vi "2DROISpectrum.vi"(4 "Zero Pad?":bool, 6 "convert output to dB?":bool, 7 "FFT size":u16(ring) items=["next 2^n", "8", "16", "32", "64", "128", "256", "512"], 8 "Cal File":dbl[](array[numeric]) format="%.2f", 9 "Array Subset":T1 {"length of y" format="%.2f"; "y start" format="%.2f"; "length of x" format="%.2f"; "x start" format="%.2f"}, 10 "freq (MHz)":dbl format="%.2f", 11 "2-D data array":i16[][](array[numeric])) -> (0 "Length of padded array":i32, 1 "df (MHz)":dbl format="%.2f", 3 "power spectrum in dB":dbl[][](array[numeric]) format="%.2f")   [LabVIEW 2022 SP3]
uses:
  <vilib>/Analysis/4window.llb/Hamming Window (DBL).vi
  <vilib>/Analysis/2dsp.llb/Real FFT.vi
  <vilib>/Analysis/2dsp.llb/Complex FFT.vi
  <vilib>/Analysis/4window.llb/AllCosWindow (DBL).vi
  <vilib>/Analysis/NI_AALPro.lvlib
panel:
  # "Columns represent scan line"
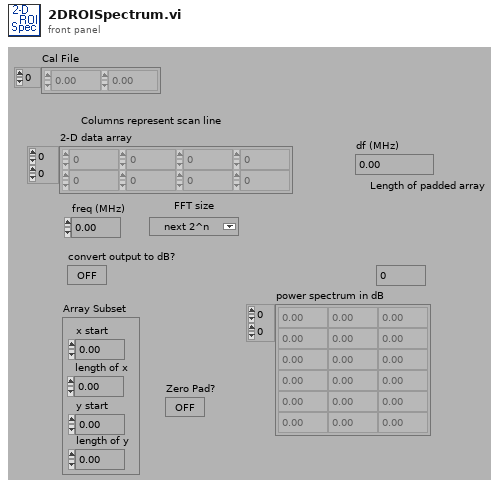
[diagram p1: front panel]
types:
  T1 = cluster{"x start":dbl, "length of x":dbl, "y start":dbl, "length of y":dbl}
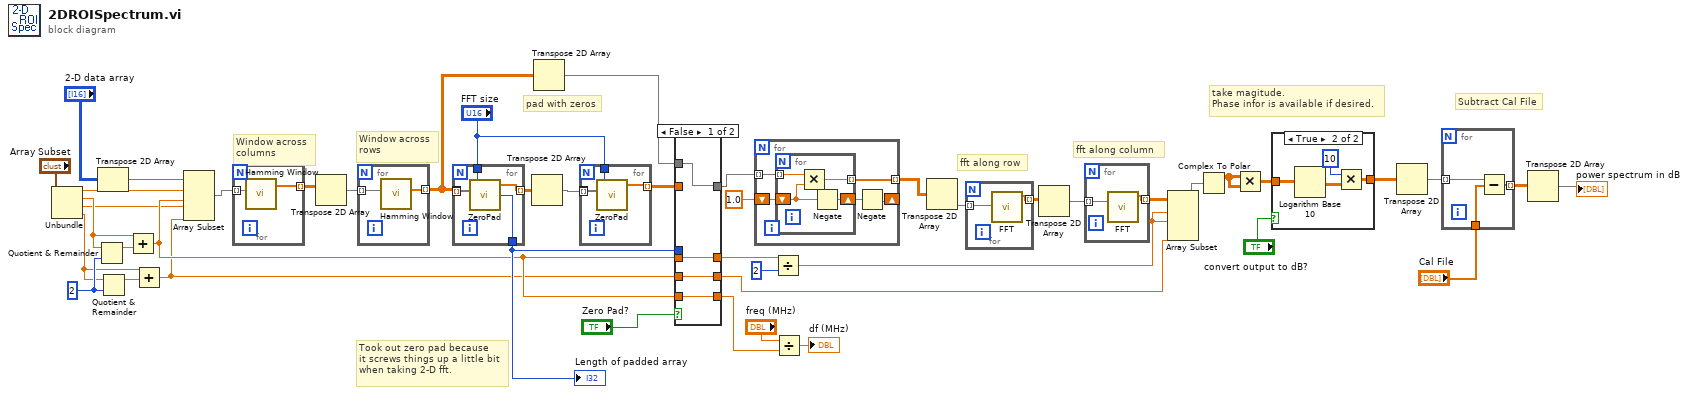
[diagram p0: block diagram]
diagram:
  w25 = 2
  # "Took out zero pad because\nit screws things up a little bit\nwhen taking 2-D fft."
  # "Subtract Cal File"
  # "take magitude.\nPhase infor is available if desired."
  # "pad with zeros"
  # "Window across\nrows"
  # "Window across\ncolumns"
  # "fft along column"
  # "fft along row"
  n1 = Unbundle("Array Subset") -> ("x start"=w6:dbl, "length of x"=w23:dbl, "y start"=w4:dbl, "length of y"=w21:dbl)
  n2 = Quotient & Remainder(x=w23, y=w25) -> (x-y*floor(x/y)=w24:dbl)  [unwired: 1 out]
  n3 = Transpose 2D Array(2D array="2-D data array") -> (transposed array=w1:i16[][])
  n4 = Quotient & Remainder(x=w21, y=w25) -> (x-y*floor(x/y)=w22:dbl)  [unwired: 1 out]
  n5 = Add(x=w23, y=w24) -> (x+y=w5:dbl)
  n6 = Add(x=w21, y=w22) -> (x+y=w3:dbl)
  n7 = Array Subset(array=w1, index (row)=w6, length (row)=w5, index (col)=w4, length (col)=w3) -> (w2:i16[][])
  n8 = for {
    tunnel: w2 -> [w48] mode=indexing
    tunnel: [w47] -> w38 mode=indexing
    n9 = call-poly <vilib>:"Hamming Window.vi"("X"=w48) -> ("Windowed X"=w47:dbl[])  [unwired: 1 out]
  }
  n10 = Transpose 2D Array(2D array=w38) -> (transposed array=w39:dbl[][])
  n11 = for {
    tunnel: [w50] -> w20 mode=indexing
    tunnel: w39 -> [w49] mode=indexing
    n12 = call-poly <vilib>:"Hamming Window.vi"("X"=w49) -> ("Windowed X"=w50:dbl[])  [unwired: 1 out]
  }
  n13 = for {
    tunnel: [w54] -> _ mode=indexing
    tunnel: [w51] -> w37 mode=indexing
    tunnel: w20 -> [w54] mode=indexing
    tunnel: "FFT size" -> [w53]
    tunnel: [w52] -> w13
    n14 = call "ZeroPad.vi"("Input Array"=w54, "FFT size"=w53) -> ("Length of padded array"=w52:i32, "Ouput Array"=w51:dbl[])  [unwired: 3 out]
  }
  "Length of padded array" <- w13
  n15 = Transpose 2D Array(2D array=w37) -> (transposed array=w42:dbl[][])
  n16 = Transpose 2D Array(2D array=w20) -> (transposed array=w16:dbl[][])
  n17 = for {
    tunnel: [w57] -> _ mode=indexing
    tunnel: [w56] -> w17 mode=indexing
    tunnel: w42 -> [w57] mode=indexing
    tunnel: "FFT size" -> [w55]
    n18 = call "ZeroPad.vi"("Input Array"=w57, "FFT size"=w55) -> ("Ouput Array"=w56:dbl[])  [unwired: 4 out]
  }
  n19 = case shown="False" "Zero Pad?" {
    tunnel: [w61 w63] -> w9
    tunnel: w17 -> [_ w63]
    tunnel: w16 -> [w61 _]
    tunnel: [w60 w62] -> w15
    tunnel: w5 -> [w60 _]
    tunnel: [w59 w62] -> w14
    tunnel: w3 -> [w59 _]
    tunnel: w13 -> [_ w62]
    tunnel: [w58 w62] -> w12
    tunnel: w5 -> [w58 _]
    frame False {
    }
    frame True {
    }
  }
  n20 = for {
    shift-right: [w64] -> _
    shift-left: 1.0 -> [w68]
    tunnel: [w67] -> w8 mode=indexing
    tunnel: w9 -> [w66] mode=indexing
    n21 = for {
      shift-right: [w72] -> w65
      shift-left: w68 -> [w71]
      tunnel: [w70] -> w67 mode=indexing
      tunnel: w66 -> [w69] mode=indexing
      n22 = Multiply(x=w69, y=w71) -> (x*y=w70:dbl)
      n23 = Negate(x=w71) -> (-x=w72:dbl)
    }
    n24 = Negate(x=w65) -> (-x=w64:dbl)
  }
  n25 = Divide(x=w15, y=2) -> (x/y=w33:dbl)
  n26 = Divide(x="freq (MHz)", y=w12) -> (x/y=→"df (MHz)":dbl)
  n27 = Transpose 2D Array(2D array=w8) -> (transposed array=w32:dbl[][])
  n28 = for {
    tunnel: w32 -> [w73] mode=indexing
    tunnel: [w74] -> w36 mode=indexing
    n29 = call-poly <vilib>:"FFT.vi"("X"=w73) -> ("FFT {X}"=w74:cdb[])  [unwired: 2 in, 8 out]
  }
  n30 = Transpose 2D Array(2D array=w36) -> (transposed array=w34:cdb[][])
  n31 = for {
    tunnel: w34 -> [w76] mode=indexing
    tunnel: [w75] -> w30 mode=indexing
    n32 = call-poly <vilib>:"FFT.vi"("X"=w76) -> ("FFT {X}"=w75:cdb[])  [unwired: 2 in, 8 out]
  }
  n33 = Array Subset(array=w30, index (row)=w33, length (row)=w33, length (col)=w14) -> (w19:cdb[][])  [unwired: 1 in]
  n34 = Complex To Polar(r * e^(i*theta)=w19) -> (r=w18:dbl[][])  [unwired: 1 out]
  n35 = Multiply(x=w18, y=w18) -> (x*y=w35:dbl[][])
  n36 = case shown="True" "convert output to dB?" {
    tunnel: [w77 w80] -> w31
    tunnel: w35 -> [w77 w78]
    frame False {
    }
    frame True {
      n37 = Logarithm Base 10(1:w78) -> (0:w81:dbl[][])
      n38 = Multiply(x=10, y=w81) -> (x*y=w80:dbl[][])
    }
  }
  n39 = Transpose 2D Array(2D array=w31) -> (transposed array=w29:dbl[][])
  n40 = for {
    tunnel: w29 -> [w84] mode=indexing
    tunnel: "Cal File" -> [w83]
    tunnel: [w82] -> w27 mode=indexing
    n41 = Subtract(x=w84, y=w83) -> (x-y=w82:dbl[])
  }
  n42 = Transpose 2D Array(2D array=w27) -> (transposed array=→"power spectrum in dB":dbl[][])
